vi "init.vi"(8 "error in (no error)":errorcluster, 11 "EncoderReader in":refnum<class "EncoderReader.lvclass">) -> (0 "error out":errorcluster, 3 "EncoderReader out":refnum<class "EncoderReader.lvclass">)   [LabVIEW 2013, in "EncoderReader.lvclass"]
uses:
  EncoderReader.lvclass
  Configuration/Encoder Reader.ctl
  <userlib>/Common/SerialProtocols/Configuration/SerialConfig.ctl
  <userlib>/Common/SerialProtocols/Configuration/SerialProtocol.ctl
  <userlib>/Common/SerialProtocols/Configuration/ProtocolParameters.ctl
  <userlib>/Common/SerialProtocols/Configuration/SerialMessageParameters.ctl
  EncoderReader.lvclass/EncoderReader.ctl
  ConfigurationThisComponent/ConfigurationThisComponent.lvclass
  <userlib>/Common/SerialProtocols/SerialProtocols.lvlib
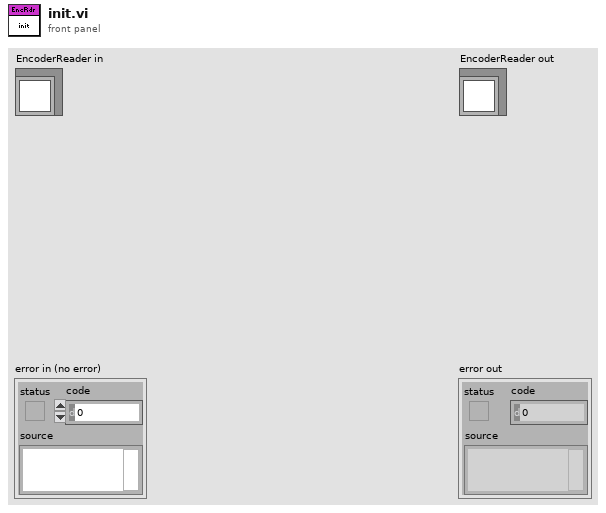
[diagram p1: front panel]
types:
  T1 = typedef "Encoder Reader.ctl" = cluster{"Serial":T2}
  T2 = typedef "SerialProtocols.lvlib/SerialConfig.ctl" = cluster{"Serial Protocol":T3, "Protocol Parameters":T4, "Serial Message Parameters":T5}
  T3 = typedef "SerialProtocols.lvlib/SerialProtocol.ctl" = enum16{"RS232", "RS485", "SerialSimulator"}
  T4 = typedef "SerialProtocols.lvlib/ProtocolParameters.ctl" = cluster{"VISA resource name":refnum<visa-resource-name>, "Baud Rate":u32, "Data Bits":u16, "Parity":enum16{"None", "Odd", "Even", "Mark", "Space"}, "Flow Control":u16, "Stop Bits":u16, "Timeout (ms)":u32}
  T5 = typedef "SerialProtocols.lvlib/SerialMessageParameters.ctl" = cluster{"Byte Count":u32, "Enable Termination Character":bool, "Termination Char":u8}
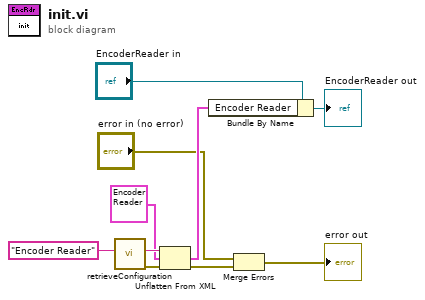
[diagram p0: block diagram]
diagram:
  n1 = call "retrieveConfiguration.vi"("configName"="Encoder Reader") -> ("error out"=w8:errorcluster, "xmlConfig"=w9:string)  [unwired: 8 in, 1 out]
  n2 = Unflatten From XML(xml string=w9, type=T1 {"Serial"={"Serial Protocol"=enum."RS485", "Protocol Parameters"={"VISA resource name"="", "Baud Rate"=9600, "Data Bits"=8, "Parity"=enum."None", "Flow Control"=0, "Stop Bits"=10, "Timeout (ms)"=10000}, "Serial Message Parameters"={"Byte Count"=200, "Enable Termination Character"=FALSE, "Termination Char"=200}}} ("Encoder Reader"), error in (no error)=w8) -> (value=w4:T1, error out=w3:errorcluster)
  n3 = Bundle By Name(cluster="EncoderReader in", "Encoder Reader"=w4) -> (→"EncoderReader out":refnum<class "EncoderReader.lvclass">)
  n4 = Merge Errors("error in (no error)", w3) -> (→"error out":errorcluster)
